vi "add_linker_info_array.vi"(6 "include all? (false: use links to include array)":bool, 8 "error in":errorcluster, 9 "links to include":u32[](array[numeric]), 10 "Linker Info":T1(array[cluster]), 11 "HierarchyGraph in":refnum<class "HierarchyGraph.lvclass">) -> (0 "error out":errorcluster, 3 "HierarchyGraph out":refnum<class "HierarchyGraph.lvclass">)   [LabVIEW 2020]
uses:
  HierarchyGraph.lvclass
  C:/Projects/labview-project-load-tools/source/submodules/graph-api-labview/source/api/Graph/Graph.lvclass
  VINode/HierarchyNode.lvclass
  C:/Projects/labview-project-load-tools/source/submodules/graph-api-labview/source/api/Node/Node.lvclass
  api/Node/Node.lvclass/Node.ctl
  api/Graph/Graph.lvclass/Graph.ctl
  7f46277b-0bd0-4fe3-8d88-c59fe5d109fd.vi
  api/Node/get_id.vi
  b52b454a-04d4-425c-933c-41725125f972.vi/7c7783df-fd5a-49d9-9b7a-63cc9fb0e4e5.vi
  api/Graph/Graph.lvclass
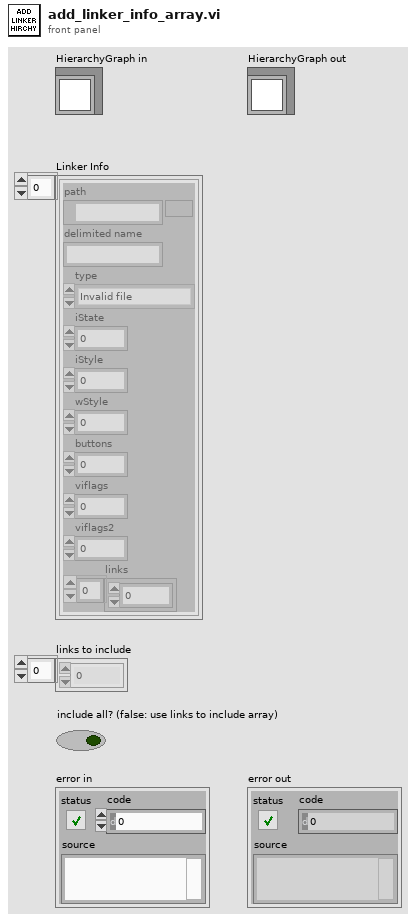
[diagram p1: front panel]
types:
  T1 = cluster{"path":path, "delimited name":string, "type":enum32{"Invalid file", "Unknown type", "Instrument", "Control", "Polymorphic VI", "Project", "Library", "LVClass", "XControl", "XNode", "Shared library", ".NET assembly", "ActiveX interface", "CIN", "Run-time menu", "Palette menu", "Help file", "LLB", "XNode Edit Dependency", "Class Private Data Control", "Statechart", "MathScript .m file", "Ladder Diagram"}, "iState":u32, "iStyle":u16, "wStyle":u16, "buttons":u16, "viflags":u32, "viflags2":u32, "links":u32[]}[]
  T2 = cluster{"path":path, "delimited name":string, "type":enum32{"Invalid file", "Unknown type", "Instrument", "Control", "Polymorphic VI", "Project", "Library", "LVClass", "XControl", "XNode", "Shared library", ".NET assembly", "ActiveX interface", "CIN", "Run-time menu", "Palette menu", "Help file", "LLB", "XNode Edit Dependency", "Class Private Data Control", "Statechart", "MathScript .m file", "Ladder Diagram"}, "iState":u32, "iStyle":u16, "wStyle":u16, "buttons":u16, "viflags":u32, "viflags2":u32, "links":u32[]}
  T3 = enum32{"Invalid file", "Unknown type", "Instrument", "Control", "Polymorphic VI", "Project", "Library", "LVClass", "XControl", "XNode", "Shared library", ".NET assembly", "ActiveX interface", "CIN", "Run-time menu", "Palette menu", "Help file", "LLB", "XNode Edit Dependency", "Class Private Data Control", "Statechart", "MathScript .m file", "Ladder Diagram"}
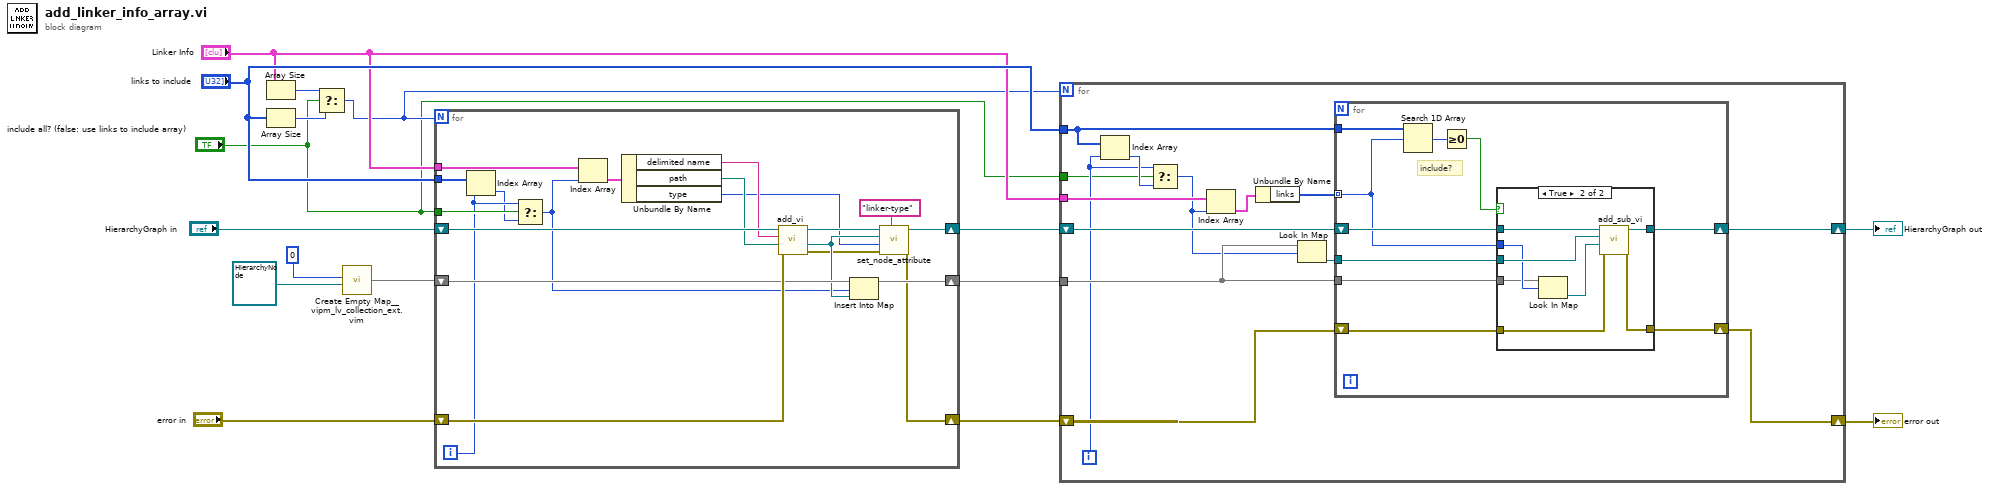
[diagram p0: block diagram]
diagram:
  n1 = Array Size(array="Linker Info") -> (size(s)=w4:i32)
  n2 = Array Size(array="links to include") -> (size(s)=w3:i32)
  n3 = Select(t=w4, s="include all? (false: use links to include array)", f=w3) -> (s? t:f=w2:i32)
  n4 = call "Create Empty Map__vipm_lv_collection_ext.vim"("value type"=refnum<class "HierarchyNode.lvclass"> refnum ("VINode out"), "key type"=u32 0) -> ("empty map"=w7:map{u32, refnum<class "HierarchyNode.lvclass">})  [unwired: 8 in]
  n5 = for {
    N: w2 -> [_]
    tunnel: "Linker Info" -> [w36]
    shift-right: [w27] -> w14
    shift-left: "HierarchyGraph in" -> [w35]
    shift-right: [w22] -> w13
    shift-left: "error in" -> [w34]
    tunnel: "links to include" -> [w21]
    shift-right: [w30] -> w10
    shift-left: w7 -> [w29]
    tunnel: "include all? (false: use links to include array)" -> [w20]
    i -> [w19]
    n6 = Index Array(array=w21, index=w19) -> (element=w18:u32)
    n7 = Select(t=w19, s=w20, f=w18) -> (s? t:f=w17:u32)
    n8 = Index Array(array=w36, index=w17) -> (element=w33:T2)
    n9 = Unbundle By Name(w33) -> ("delimited name"=w32:string, "path"=w31:path, "type"=w24:T3)
    n10 = call "add_vi.vi"("error in (no error)"=w34, "Path"=w31, "vi_name"=w32, "VIGraph in"=w35) -> ("error out"=w23:errorcluster, "VINode out"=w25:refnum<class "HierarchyNode.lvclass">, "VIGraph out"=w28:refnum<class "HierarchyGraph.lvclass">)  [unwired: 4 in, 1 out]
    n11 = Insert Into Map(map in=w29, key=w17, value=w25) -> (map out=w30:map{u32, refnum<class "HierarchyNode.lvclass">})  [unwired: 2 out]
    n12 = call "set_node_attribute.vi"("name"="linker-type" ("attribute-name"), "error in (no error)"=w23, "value"=w24, "node"=w25, "graph"=w28) -> ("error out"=w22:errorcluster, "graph-out"=w27:refnum<class "HierarchyGraph.lvclass">)  [unwired: 4 in, 1 out]
  }
  n13 = for {
    N: w2 -> [_]
    tunnel: "Linker Info" -> [w50]
    shift-right: [w48] -> w12
    shift-left: w14 -> [w49]
    shift-right: [w42] -> w11
    shift-left: w13 -> [w43]
    tunnel: w10 -> [w44]
    tunnel: "links to include" -> [w40]
    tunnel: "include all? (false: use links to include array)" -> [w38]
    i -> [w39]
    n14 = Index Array(array=w40, index=w39) -> (element=w41:u32)
    n15 = Select(t=w39, s=w38, f=w41) -> (s? t:f=w37:u32)
    n16 = Index Array(array=w50, index=w37) -> (element=w47:T2)
    n17 = Unbundle By Name(w47) -> ("links"=w46:u32[])
    n18 = Look In Map(map=w44, key=w37) -> (value=w45:refnum<class "HierarchyNode.lvclass">)  [unwired: 1 in, 1 out]
    n19 = for {
      shift-right: [w59] -> w48
      shift-left: w49 -> [w60]
      tunnel: w46 -> [w53] mode=indexing
      tunnel: w45 -> [w58]
      tunnel: w44 -> [w57]
      shift-right: [w55] -> w42
      shift-left: w43 -> [w56]
      tunnel: w40 -> [w54]
      # "include?"
      n20 = Search 1D Array(1D array=w54, element=w53) -> (index of element=w52:i32)  [unwired: 1 in]
      n21 = Greater Or Equal To 0?(x=w52) -> (x >= 0?=w51:bool)
      n22 = case shown="True" w51 {
        tunnel: w60 -> [w62 w70]
        tunnel: [w62 w69] -> w59
        tunnel: w58 -> [_ w68]
        tunnel: w53 -> [_ w67]
        tunnel: w57 -> [_ w66]
        tunnel: w56 -> [w61 w64]
        tunnel: [w61 w63] -> w55
        frame False {
        }
        frame True {
          n23 = Look In Map(map=w66, key=w67) -> (value=w65:refnum<class "HierarchyNode.lvclass">)  [unwired: 1 in, 1 out]
          n24 = call "add_sub_vi.vi"("error in (no error)"=w64, "SubVI"=w65, "VI"=w68, "VIHierarchyGraph in"=w70) -> ("error out"=w63:errorcluster, "VIHierarchyGraph out"=w69:refnum<class "HierarchyGraph.lvclass">)  [unwired: 6 in]
        }
      }
    }
  }
  "error out" <- w11
  "HierarchyGraph out" <- w12
